vi "Init Transport.vi"() -> (2 "Transport":refnum<class "Transport.lvclass">)   [LabVIEW 2025, in "jettl.lvlib" / "Notifier Transport.lvlib"]
uses:
  Notifier Transport.lvlib
  Notifier Transport/Notifier Transport.lvclass
  Transport/Transport.lvclass
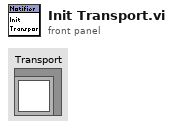
[diagram p1: front panel]
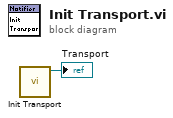
[diagram p0: block diagram]
diagram:
  n1 = call "Init Transport.vi"() -> ("Notifier Transport out"=→"Transport":refnum<class "Notifier Transport.lvclass">)  [unwired: 11 in]
